vi "MCCMSG Get Secondary Signal.vi"(8 "error in (no error)":errorcluster, 9 "pnError":i32, 10 "puSignalID":u32, 11 "hMCCmsg":i32) -> (0 "error out":errorcluster, 1 "pnError out":i32, 2 "puSignalID out":u32, 3 "function return":i32)   [LabVIEW 2012, in "MultiClamp 700B Controls.lvlib" / "AxMultiClampMsg.lvlib"]
doc: "AXMCCMSG BOOL WINAPI MCCMSG_GetSecondarySignal(HMCCMSG hMCCmsg, UINT *puSignalID, int *pnError);"
uses:
  AxMultiClampMsg.lvlib
  AxMultiClampMsg.dll
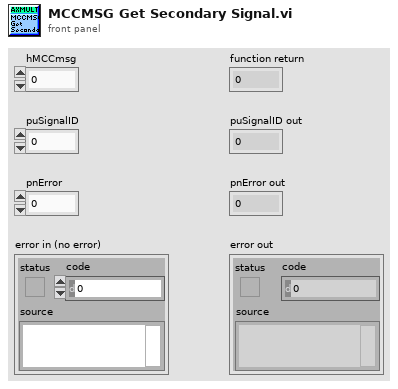
[diagram p1: front panel]
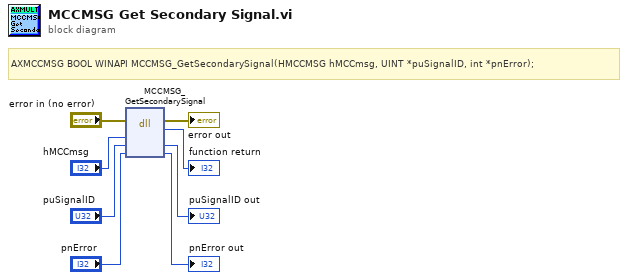
[diagram p0: block diagram]
diagram:
  # "AXMCCMSG BOOL WINAPI MCCMSG_GetSecondarySignal(HMCCMSG hMCCmsg, UINT *puSignalID, int *pnError);"
  n1 = dll-call lib="C:/Users/LAA12/Desktop/Rita/Multiclamp 700B VIs/AxMultiClampMsg/AxMultiClampMsg.*" fn="MCCMSG_GetSecondarySignal"(error in="error in (no error)", "hMCCmsg"="hMCCmsg", "puSignalID"="puSignalID", "pnError"="pnError") -> (error out=→"error out":errorcluster, →"function return":i32, "puSignalID"=→"puSignalID out":u32, "pnError"=→"pnError out":i32)  [unwired: 3 in, 1 out]
